vi "KundtsTube.vi"() -> ()   [LabVIEW 2015]
uses:
  <vilib>/imath/engines/lvmath2/RunTimeEngine/Managers/WorkSpace/UID Generator.vi
  <vilib>/imath/engines/lvmath2/RunTimeEngine/RunTimeType/NIMS_RunTimeType_From StrictType (excl LVString).vi
  <instcachedir>/0/NIMS_RunTimeType_From StrictType (excl LVString)_EB1C38A9BC5048DA9ABDA8F781E54D21.lvgen/NIMS_RunTimeType_From StrictType (excl LVString)_EB1C38A9BC5048DA9ABDA8F781E54D21_000.vi
  <vilib>/imath/engines/lvmath2/RunTimeEngine/LocalVariableDefStatement/MC_LocalVariableDefStatement_Display.vi
  <vilib>/imath/engines/lvmath2/RunTimeEngine/Managers/SymbolTable/Clear UID.vi
  <vilib>/imath/engines/lvmath2/RunTimeEngine/NodeEndStatement/NIMS_NodeEndStatement_Output.vi
  <instcachedir>/0/NIMS_NodeEndStatement_Output_53EC0D466D134D7ABD903AC30B43404B.lvgen/NIMS_NodeEndStatement_Output_53EC0D466D134D7ABD903AC30B43404B_009.vi
  <vilib>/imath/engines/lvmath2/RunTimeEngine/ErrorHandling/NIMS_Finalize Error.vi
  <vilib>/Utility/file.llb/Write Delimited Spreadsheet (DBL).vi
  <vilib>/imath/engines/lvmath2/RunTimeEngine/Managers/SymbolTable/NIMS_WorkSpace.lvlib
panel:
  out "Waveform Graph":dbl[](graph)=[0.003133375259297034, 0.003237727419167467, 0.0028050789609904646, 0.04361870281699251, 0.08811537536201913, 0.7410766535452404, 0.14407203227125412, 0.2403300501886206, 0.23573112236420785, 0.12277661272428483, 0.484853183728046, 0.10367983736429286, 0.09055596802669953, 0.2923720986893444, 0.059819349672162896, 0.10255100585324274, 0.07624556825296276, 0.04607990694738208, 0.3673763555454811, 0.04045942831966469, 0.048329467868846544, 0.08430397522380657, 0.03185011495589433, 0.08015602125208923, 0.03688543181512353, 0.02914746867151676, 0.2411755441992505, 0.026206620216184848, 0.03478751294981375, 0.051413970047189915, 0.02195875622551037, 0.060551460840002395, 0.027515935000052616, 0.022082127887283205, 0.17835009783936048, 0.02021022180373137, 0.027043763410133533, 0.0424368820481907, 0.018049871137295424, 0.05176098629453348, 0.02356960762017828, 0.02076419435468337, 0.12404982906010485, 0.019703744990745897, 0.03058605689958258, 0.03530784140830944, 0.020090242117358794, 0.0802504505471437, 0.025472163526541535, 0.024498518998926192, 0.10620225853249389, 0.025117455032383343, 0.03780968534300976, 0.0494106651018037, 0.024430345937236565, 0.05816954442200335, 0.03505250810932622, 0.0245659402517905, 0.10472531320598283, 0.0268925029772105, 0.024787261873459702, 0.10201396080311277, 0.019722452959180726, 0.028076977501401177, 0.03682435400579546, 0.015994210077392792, 0.041546690963949195, 0.01948469197374096, 0.015242056402845892, 0.07213650211081368, 0.013315850155123305, 0.0175005402877771, 0.02509453224445367, 0.011691776678458492, 0.02954539217282984, 0.014232741318400799, 0.012167655923390579, 0.054983214619929985, 0.01119499183521336, 0.015135373362837904, 0.02966620439334963, 0.010394058923786165, 0.017706853352711025, 0.016129192467571895, 0.009203321483457405, 0.02710737464011503, 0.010812618396893165, 0.009007786382306432, 0.034086437683869125, 0.008196343236628998, 0.010102856964806272, 0.015858228037389305, 0.007356028497510875, 0.014438730899677519, 0.00946530893744923, 0.01689553516946812, 0.025013815465275976, 0.007587827996567584, 0.00808537998777727, 0.019783810236316823]
  out "Gain vs Frequency":cluster{dbl[], "Array":dbl[]}(graph)={[10.0, 111.0, 212.0, 313.0, 414.0, 515.0, 615.0, 716.0, 817.0, 918.0, 1019.0, 1120.0, 1221.0, 1322.0, 1423.0, 1524.0, 1625.0, 1725.0, 1826.0, 1927.0, 2028.0, 2129.0, 2230.0, 2331.0, 2432.0, 2533.0, 2634.0, 2735.0, 2835.0, 2936.0, 3037.0, 3138.0, 3239.0, 3340.0, 3441.0, 3542.0, 3643.0, 3744.0, 3845.0, 3945.0, 4046.0, 4147.0, 4248.0, 4349.0, 4450.0, 4551.0, 4652.0, 4753.0, 4854.0, 4955.0, 5055.0, 5156.0, 5257.0, 5358.0, 5459.0, 5560.0, 5661.0, 5762.0, 5863.0, 5964.0, 6065.0, 6165.0, 6266.0, 6367.0, 6468.0, 6569.0, 6670.0, 6771.0, 6872.0, 6973.0, 7074.0, 7175.0, 7275.0, 7376.0, 7477.0, 7578.0, 7679.0, 7780.0, 7881.0, 7982.0, 8083.0, 8184.0, 8285.0, 8385.0, 8486.0, 8587.0, 8688.0, 8789.0, 8890.0, 8991.0, 9092.0, 9193.0, 9294.0, 9395.0, 9495.0, 9596.0, 9697.0, 9798.0, 9899.0, 10000.0], "Array"=[-53.090051757169725, -52.8054942933357, -54.05139813969968, -30.216845038892558, -24.10926604440991, -5.613037322290385, -19.838706309703838, -15.394138413624056, -15.561961477238766, -21.227987006874013, -9.298094922716558, -22.69641381107966, -23.871958407392317, -13.691581452990608, -27.47346621112778, -22.791501468135607, -25.366007845894334, -29.740068088388476, -11.708075925766884, -30.869905116253076, -29.326059689242243, -24.49333888477139, -32.94807987337225, -24.931576921692216, -31.673202515065185, -33.71828307300829, -15.363634613463004, -34.642079656827974, -32.18183233643434, -28.788677152585297, -36.17814520801417, -27.36780745227759, -34.21861445944282, -36.12948154182078, -17.984832918242603, -36.898878359655846, -34.3689573987291, -30.455430604273083, -37.8808178424005, -28.730249094079014, -35.563252905058576, -36.663998251432986, -21.138376553569064, -37.11932439356796, -33.299830114319384, -32.05287661252365, -36.950596543129, -24.921350370095, -34.88898327351699, -35.22750333876545, -22.487624902753502, -35.01078728828637, -31.458238694162006, -29.13388595996899, -35.25170762284507, -27.716386707416415, -32.11591798757932, -35.203632131819404, -22.609266598714868, -34.41767544910013, -35.12572885567203, -22.837107759663702, -37.11108137903334, -34.04329287688218, -31.68759721793051, -38.93104403666594, -30.63957116479095, -37.216429064983735, -39.349428668851665, -25.84719836439025, -40.522921969766756, -38.149270822481746, -35.018717857490415, -41.652689728233625, -33.600504776797194, -39.944528835074394, -41.30616155159502, -28.20569740695476, -42.02982433317238, -39.41043718264095, -33.56506026486395, -42.67459646656694, -38.047472146697345, -38.85804747018318, -43.731408101889315, -34.348550796120236, -42.331682437196996, -43.91793838803434, -32.35866763231292, -44.737897217174485, -42.921415869903115, -39.005206784494185, -45.677431895814536, -39.81971950954182, -43.48760408797081, -38.454860902766164, -35.04670112472353, -45.40795040473806, -44.856291252330855, -37.08410120307653]}
  in  "?":enum32{"Single", "Sweep"}(tab)=enum."Sweep"
  in  "Frequency":dbl=1000.0
  in  "Dwell time, sec":dbl=1.0 format="%#_2f"
  out "Output":cluster{"RMS":dbl, "Frequency ":dbl}={"RMS"=0.003004852978353948, "Frequency "=212.0}
  in  "?":bool
  in  "Amplitude":dbl=2.0
  in  "?":T1={"Minimum"=10.0, " Maximum"=10000.0, "Spacing"=enum."Linear", " # of Steps"=100.0}
  in  "Sampling Rate (Hz)":dbl=100000.0
  in  "# of Samples":dbl=100000.0
  # "This will evaluate only at the selected frequency."
  # "This will sweep from min to max, pausing by the dwell time after each increment"
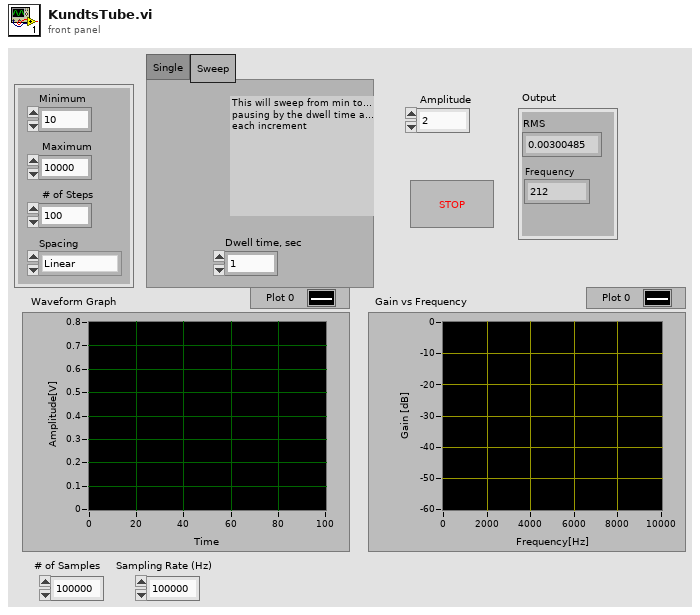
[diagram p1: front panel]
types:
  T1 = cluster{"Minimum":dbl, " Maximum":dbl, "Spacing":enum16{"Logarithmic", "Linear"}, " # of Steps":dbl}
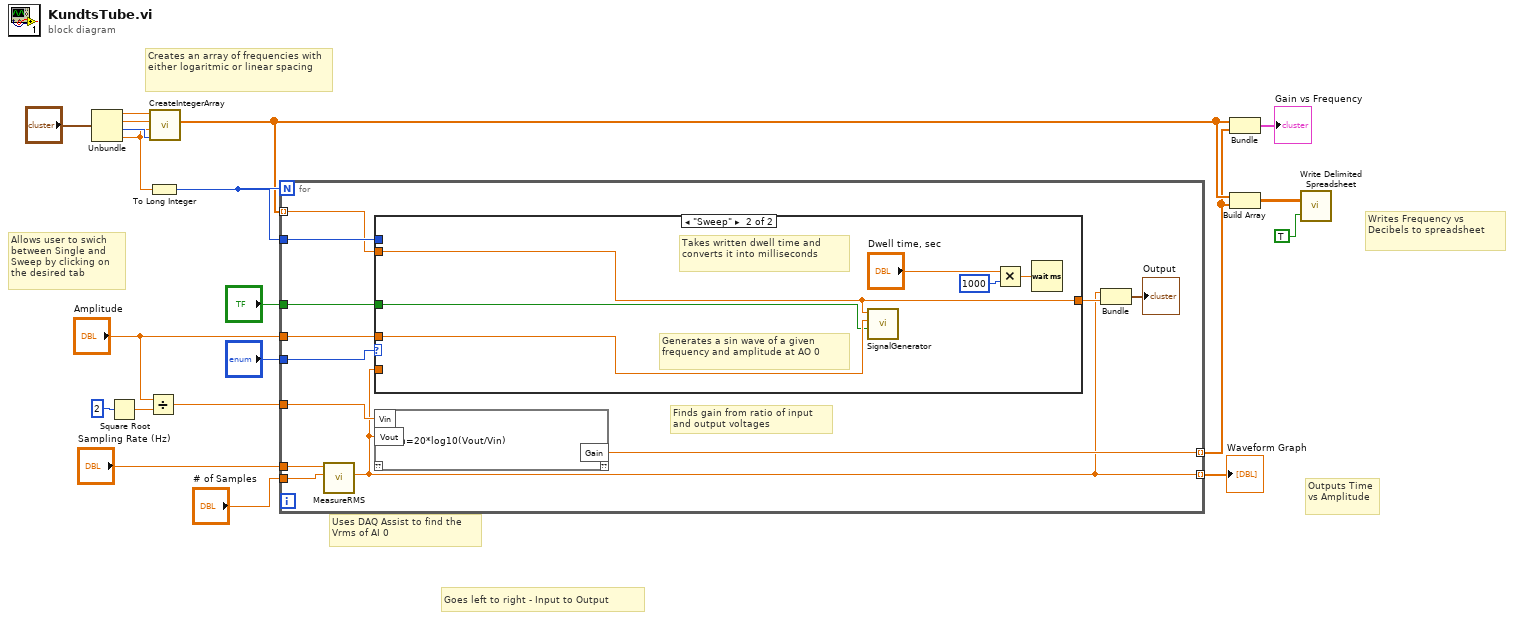
[diagram p0: block diagram]
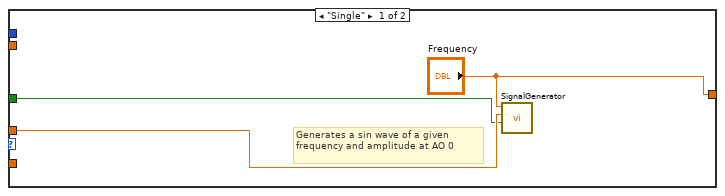
[diagram p2: hidden frame]
diagram:
  # "Outputs Time vs Amplitude"
  # "Allows user to swich between Single and Sweep by clicking on the desired tab"
  # "Uses DAQ Assist to find the Vrms of AI 0"
  # "Creates an array of frequencies with either logaritmic or linear spacing"
  # "Writes Frequency vs Decibels to spreadsheet"
  # "Goes left to right - Input to Output"
  n1 = Unbundle("?") -> ("Minimum"=w19:dbl, "Maximum"=w18:dbl, "Spacing"=w17:enum16{"Logarithmic", "Linear"}, "# of Steps"=w16:dbl)
  n2 = Square Root(x=2) -> (sqrt(x)=w12:dbl)
  n3 = Divide(x="Amplitude", y=w12) -> (x/y=w7:dbl)
  n4 = To Long Integer(number=w16) -> (32bit integer=w10:i32)
  n5 = call "CreateIntegerArray.vi"("Enum"=w17, "# of Points"=w16, "Maximum"=w18, "Minimum"=w19) -> ("Array"=w4:dbl[])  [unwired: 7 in]
  n6 = for {
    N: w10 -> [_]
    tunnel: "?" -> [w32]
    tunnel: "?" -> [w31]
    tunnel: "Amplitude" -> [w30]
    tunnel: w10 -> [w29]
    tunnel: w4 -> [w23] mode=indexing
    tunnel: "# of Samples" -> [w26]
    tunnel: "Sampling Rate (Hz)" -> [w25]
    tunnel: w7 -> [w24]
    tunnel: [w22] -> w3 mode=indexing
    tunnel: [w21] -> w6 mode=indexing
    # "Finds gain from ratio of input and output voltages"
    n7 = call "MeasureRMS.vi"("# of Samples"=w26, "Sampling Rate (Hz)"=w25) -> ("RMS"=w21:dbl)  [unwired: 8 in, 1 out]
    n8 = case shown="\"Sweep\"" w32 {
      tunnel: w29 -> [_ _]
      tunnel: w23 -> [_ w80]
      tunnel: w30 -> [w76 w82]
      tunnel: w31 -> [w75 w81]
      tunnel: w21 -> [_ _]
      tunnel: ["Frequency" w80] -> w28
      frame "Single" {
        # "Generates a sin wave of a given frequency and amplitude at AO 0"
        n9 = call "SignalGenerator.vi"("stop"=w75, "Amplitude"=w76, "Frequency"="Frequency") -> ()  [unwired: 7 in, 1 out]
      }
      frame "Sweep" {
        # "Takes written dwell time and converts it into milliseconds"
        # "Generates a sin wave of a given frequency and amplitude at AO 0"
        n10 = call "SignalGenerator.vi"("stop"=w81, "Amplitude"=w82, "Frequency"=w80) -> ()  [unwired: 7 in, 1 out]
        n11 = Multiply(x="Dwell time, sec", y=1000) -> (x*y=w79:dbl)
        n12 = Wait (ms)(milliseconds to wait=w79) -> ()  [unwired: 1 out]
      }
    }
    n13 = mathscript code="Gain=20*log10(Vout/Vin)"("Vin"=w24, "Vout"=w21) -> ("Gain"=w22:cdb)  [unwired: 1 in, 1 out]
    n14 = Bundle("RMS"=w21, "Numeric"=w28) -> (→"Output":cluster{"RMS":dbl, "Numeric":dbl})  [unwired: 1 in]
  }
  "Waveform Graph" <- w6
  n15 = Bundle("Array"=w4, w3) -> (→"Gain vs Frequency":cluster{"Array":dbl[], cdb[]})  [unwired: 1 in]
  n16 = Build Array(w4, w3) -> (w1:cdb[][])
  n17 = call-poly <vilib>:"Write Delimited Spreadsheet.vi"("2D data"=w1, "transpose? (F)"=TRUE) -> ()  [unwired: 12 in, 2 out]
